vi "TipStrip position math.vi"(7 "screens":T2[](array[typedef]), 8 "height":u32, 9 "width":u32, 10 "vertical (mouse)":i32, 11 "horizontal (mouse)":i32) -> (3 "Front Panel Window:Panel Bounds":T1)   [LabVIEW 2021, in "TipStripOOPanel.lvlib"]
uses:
  TipStripOOPanel.lvlib
  tipstrip_screens.ctl
  <vilib>/Utility/miscctls.llb/LVRectTypeDef.ctl
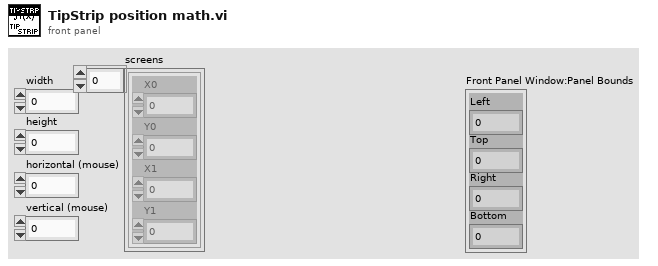
[diagram p1: front panel]
types:
  T1 = typedef "LVRectTypeDef.ctl" = cluster{"Left":i16, "Top":i16, "Right":i16, "Bottom":i16}
  T2 = typedef "TipStripOOPanel.lvlib/tipstrip_screens.ctl" = cluster{"X0":i32, "Y0":i32, "X1":i32, "Y1":i32}
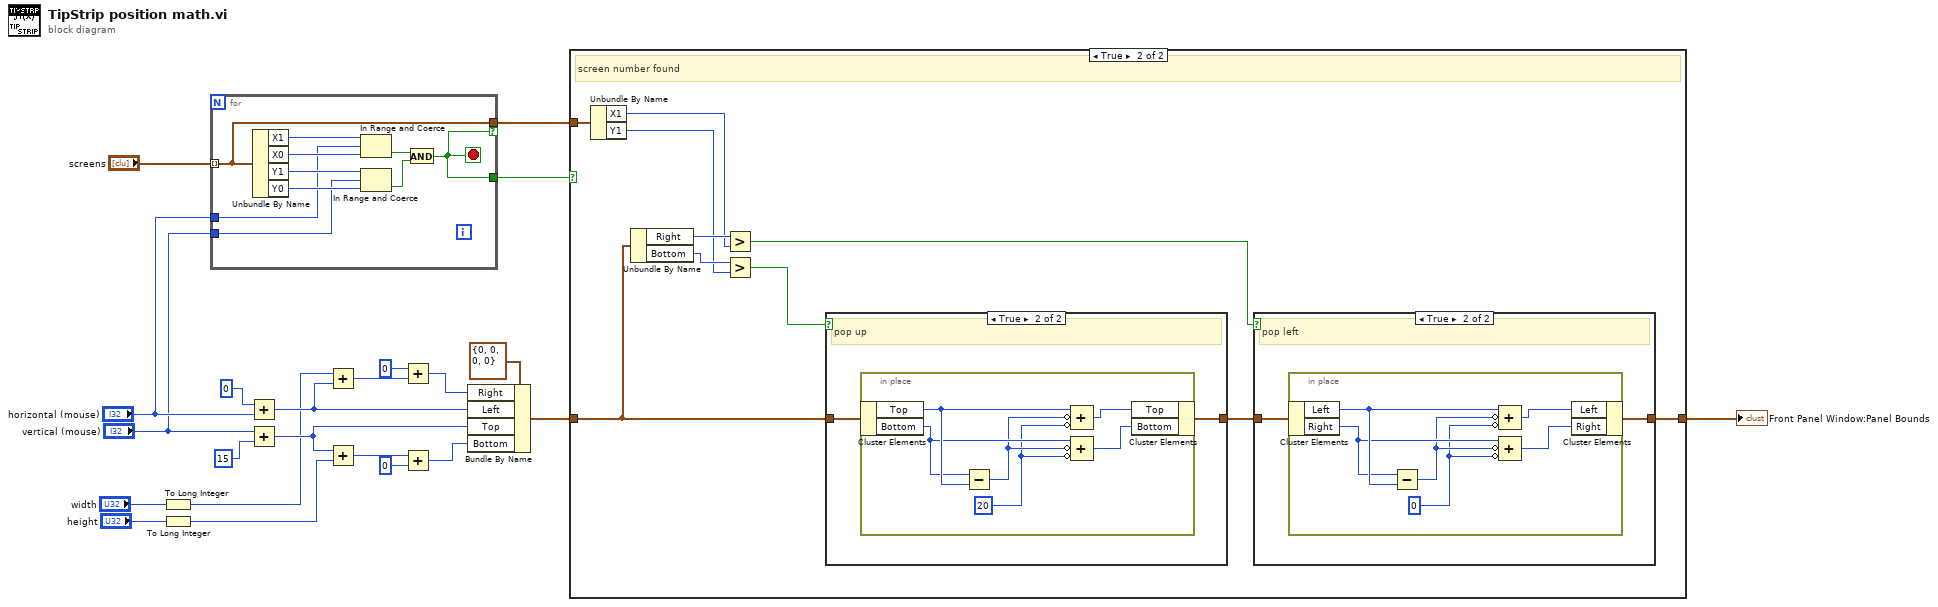
[diagram p0: block diagram]
diagram:
  n1 = To Long Integer(number="width") -> (32bit integer=w2:i32)
  n2 = To Long Integer(number="height") -> (32bit integer=w1:i32)
  n3 = for {
    tunnel: "screens" -> [w24] mode=indexing
    tunnel: [w24] -> w8 if=w23
    tunnel: "horizontal (mouse)" -> [w26]
    tunnel: "vertical (mouse)" -> [w25]
    tunnel: [w23] -> w5
    stop <- w23 stop-if-true
    n4 = Unbundle By Name(w24) -> ("X1"=w32:i32, "X0"=w31:i32, "Y1"=w30:i32, "Y0"=w29:i32)
    n5 = In Range and Coerce(upper limit=w32, x=w26, lower limit=w31) -> (In Range?=w28:bool)  [unwired: 1 out]
    n6 = In Range and Coerce(upper limit=w30, x=w25, lower limit=w29) -> (In Range?=w27:bool)  [unwired: 1 out]
    n7 = And(x=w28, y=w27) -> (x .and. y?=w23:bool)
  }
  n8 = Add(x=0, y="horizontal (mouse)") -> (x+y=w13:i32)
  n9 = Add(x="vertical (mouse)", y=15 ("x")) -> (x+y=w12:i32)
  n10 = Add(x=w2, y=w13) -> (x+y=w19:i32)
  n11 = Add(x=w12, y=w1) -> (x+y=w17:i32)
  n12 = Add(x=0 ("y"), y=w19) -> (x+y=w20:i32)
  n13 = Add(x=w17, y=0) -> (x+y=w18:i32)
  n14 = Bundle By Name(cluster=T1 {"Left"=0, "Top"=0, "Right"=0, "Bottom"=0} ("Front Panel Window:Panel Bounds"), "Right"=w20, "Left"=w13, "Top"=w12, "Bottom"=w18) -> (w7:T1)
  n15 = case shown="True" w5 {
    tunnel: w8 -> [_ w43]
    tunnel: w7 -> [w33 w38]
    tunnel: [w33 w35] -> w6
    frame False {
    }
    frame True {
      # "screen number found"
      n16 = Unbundle By Name(w43) -> ("X1"=w41:i32, "Y1"=w39:i32)
      n17 = Unbundle By Name(w38) -> ("Right"=w42:i16, "Bottom"=w40:i16)
      n18 = Greater?(x=w42, y=w41) -> (0:w34:bool)
      n19 = Greater?(x=w40, y=w39) -> (0:w37:bool)
      n20 = case shown="True" w37 {
        tunnel: w38 -> [w53 w55]
        tunnel: [w53 w54] -> w36
        frame False {
        }
        frame True {
          # "pop up"
          n21 = in-place {
            w57 = 20 ("x")
            n22 = in-place-cluster #1(w55) -> ("Top"=w61:i16, "Bottom"=w59:i16)
            n23 = Subtract(x=w59, y=w61) -> (x-y=w58:i16)
            n24 = Compound Arithmetic op=unknown(w61, invert w58, invert w57) -> (w60:i32)
            n25 = Compound Arithmetic op=unknown(w59, invert w58, invert w57) -> (w56:i32)
            n26 = in-place-cluster #1("Top"=w60, "Bottom"=w56) -> (w54:T1)
          }
        }
      }
      n27 = case shown="True" w34 {
        tunnel: w36 -> [w44 w46]
        tunnel: [w44 w45] -> w35
        frame False {
        }
        frame True {
          # "pop left"
          n28 = in-place {
            w48 = 0 ("x")
            n29 = in-place-cluster #2(w46) -> ("Left"=w52:i16, "Right"=w50:i16)
            n30 = Subtract(x=w50, y=w52) -> (x-y=w49:i16)
            n31 = Compound Arithmetic op=unknown(w52, invert w49, invert w48) -> (w51:i32)
            n32 = Compound Arithmetic op=unknown(w50, invert w49, invert w48) -> (w47:i32)
            n33 = in-place-cluster #2("Left"=w51, "Right"=w47) -> (w45:T1)
          }
        }
      }
    }
  }
  "Front Panel Window:Panel Bounds" <- w6
